vi "TCP_WRITE.vi"(2 "error in (no error)":errorcluster, 3 "connection ID":refnum<k5>, 4 "data":string) -> (0 "error out":errorcluster, 1 "connection ID out":refnum<k5>)   [LabVIEW 2023]
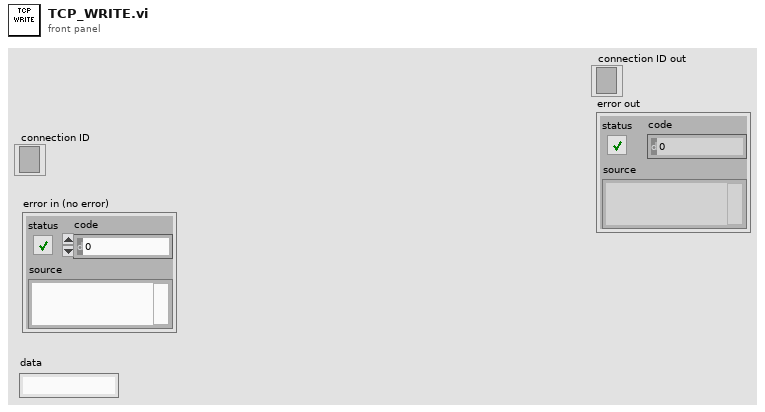
[diagram p1: front panel]
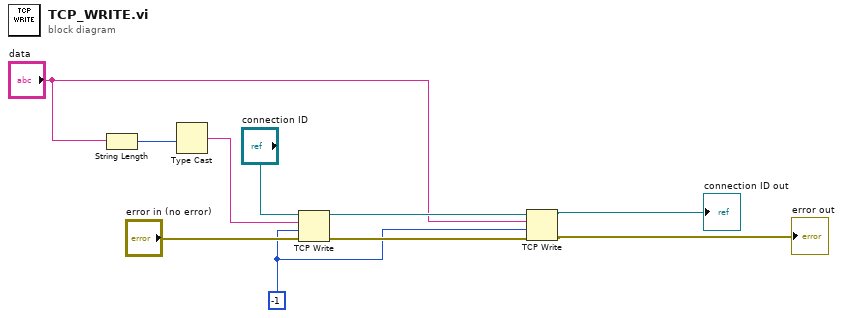
[diagram p0: block diagram]
diagram:
  w6 = -1 ("timeout ms (25000)")
  n1 = String Length(string="data") -> (length=w5:i32)
  n2 = Type Cast(x=w5) -> (*(type *) &x=w4:string)  [unwired: 1 in]
  n3 = TCP Write(connection ID="connection ID", data in=w4, error in (no error)="error in (no error)", 9:w6) -> (connection ID out=w9:refnum<k5>, error out=w10:errorcluster)  [unwired: 1 out]
  n4 = TCP Write(connection ID=w9, data in="data", error in (no error)=w10, 9:w6) -> (connection ID out=→"connection ID out":refnum<k5>, error out=→"error out":errorcluster)  [unwired: 1 out]
